vi "判斷輸贏.vi"(2 "フ":bool[][](array[boolean]), 3 "黑":bool[][](array[boolean])) -> (0 "フ墓":bool, 1 "黑贏":bool)   [LabVIEW 2014]
panel:
  out "黑贏(右上斜)":bool
  out "白贏(右上斜)":bool
  out "白贏(右下斜)":bool
  out "黑贏(右下斜)":bool
  out "フ墓(row)":bool
  out "フ墓(column)":bool
  out "黑贏(row)":bool
  out "黑贏(column)":bool
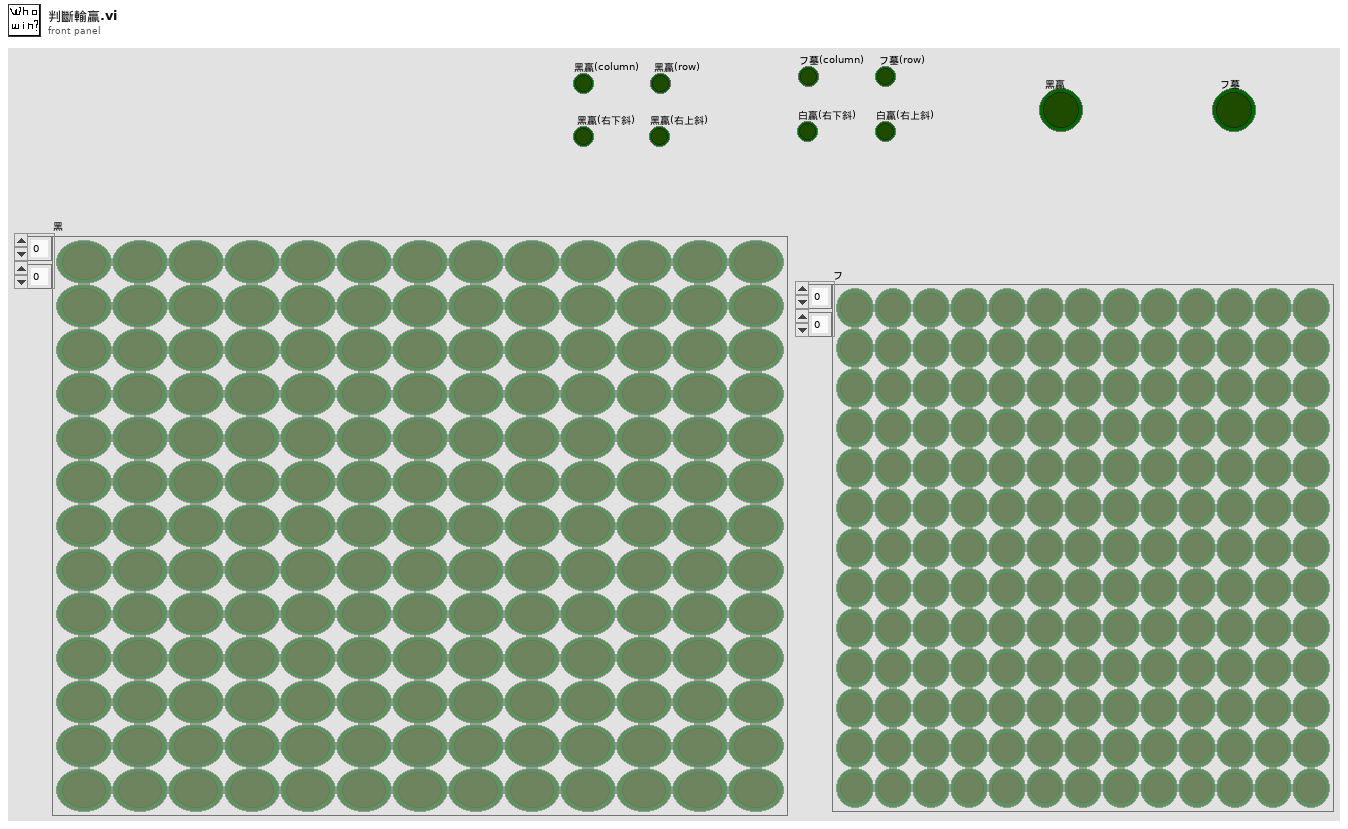
[diagram p1: front panel]
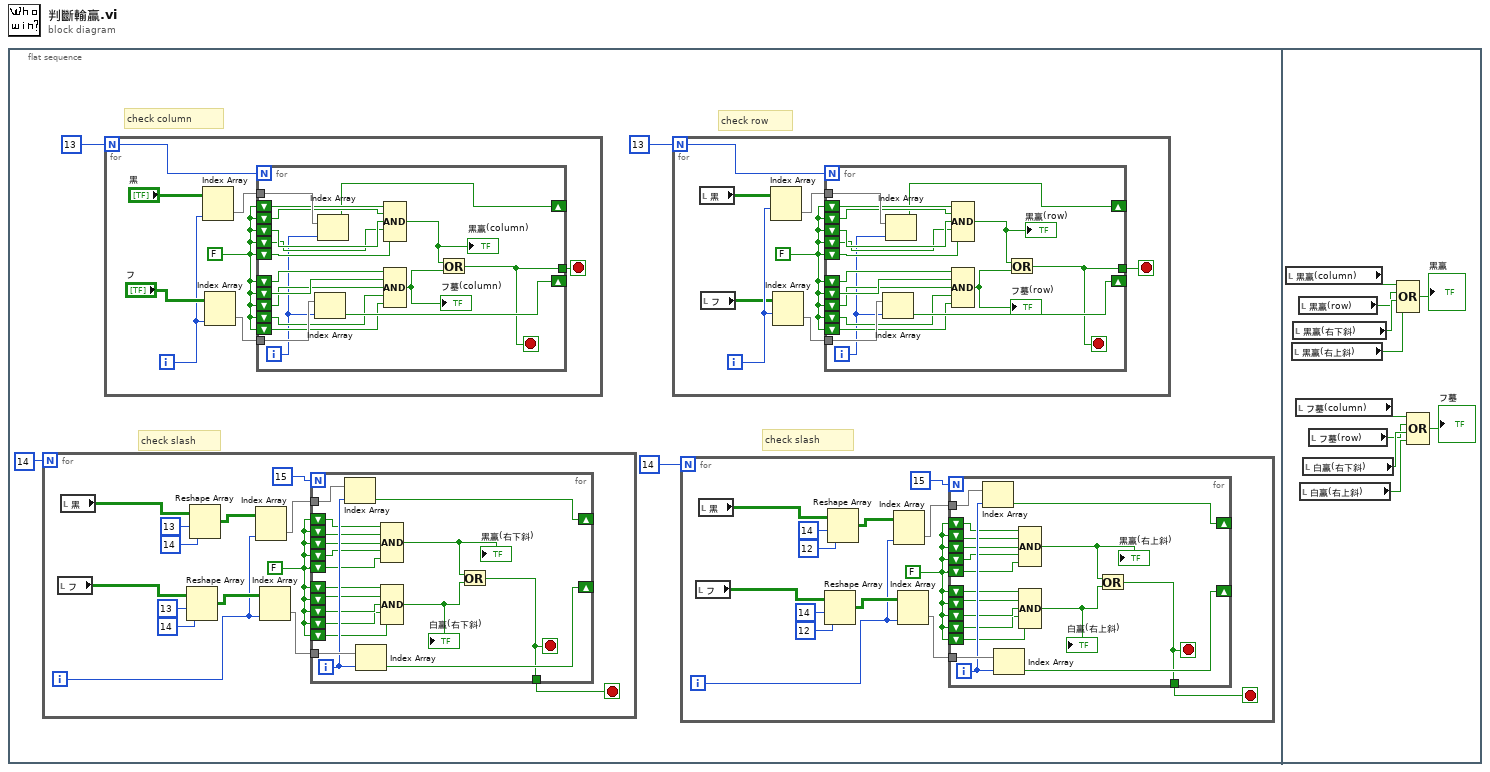
[diagram p0: block diagram]
diagram:
  n1 = flat-sequence {
    frame #0 {
      # "check slash"
      # "check slash"
      # "check row"
      # "check column"
      n2 = for {
        N: 14 -> [_]
        i -> [w42]
        stop <- w38 stop-if-true
        w39 = FALSE
        n3 = local read "フ"() -> (w48:bool[][])
        n4 = local read "黑"() -> (w47:bool[][])
        n5 = Reshape Array(w48, 13 ("dimension size"), 14 ("dimension size")) -> (w43:bool[][])
        n6 = Reshape Array(w47, 13 ("dimension size"), 14 ("dimension size")) -> (w44:bool[][])
        n7 = Index Array(array=w44, index (col)=w42) -> (element=w41:bool[])  [unwired: 1 in]
        n8 = Index Array(array=w43, index (col)=w42) -> (element=w40:bool[])  [unwired: 1 in]
        n9 = for {
          N: 15 -> [_]
          tunnel: w41 -> [w68]
          tunnel: w40 -> [w66]
          shift-right: [w67] -> _
          shift-left: w39 -> [w62]
          shift-left: w39 -> [w61]
          shift-left: w39 -> [w60]
          shift-left: w39 -> [w58]
          shift-left: w39 -> [w59]
          shift-right: [w64] -> _
          shift-left: w39 -> [w56]
          shift-left: w39 -> [w55]
          shift-left: w39 -> [w54]
          shift-left: w39 -> [w53]
          shift-left: w39 -> [w52]
          tunnel: [w63] -> w38
          i -> [w65]
          stop <- w63 stop-if-true
          n10 = Index Array(array=w68, index=w65) -> (element=w67:bool)
          n11 = Index Array(array=w66, index=w65) -> (element=w64:bool)
          n12 = Compound Arithmetic op=AND(w62, w61, w60, w59, w58) -> (w57:bool)
          "黑贏(右下斜)" <- w57
          n13 = Compound Arithmetic op=AND(w56, w55, w54, w53, w52) -> (w51:bool)
          "白贏(右下斜)" <- w51
          n14 = Or(x=w57, y=w51) -> (x .or. y?=w63:bool)
        }
      }
      n15 = for {
        N: 13 -> [w101]
        i -> [w98]
        stop <- w95 stop-if-true
        w97 = FALSE
        n16 = Index Array(array="黑", index (col)=w98) -> (element=w100:bool[])  [unwired: 1 in]
        n17 = Index Array(array="フ", index (col)=w98) -> (element=w96:bool[])  [unwired: 1 in]
        n18 = for {
          N: w101 -> [_]
          tunnel: w100 -> [w120]
          shift-right: [w114] -> _
          shift-left: w97 -> [w119]
          shift-left: w97 -> [w118]
          shift-left: w97 -> [w117]
          shift-left: w97 -> [w116]
          shift-left: w97 -> [w115]
          shift-right: [w112] -> _
          shift-left: w97 -> [w111]
          shift-left: w97 -> [w110]
          shift-left: w97 -> [w108]
          shift-left: w97 -> [w107]
          shift-left: w97 -> [w109]
          tunnel: w96 -> [w113]
          tunnel: [w104] -> w95
          i -> [w103]
          stop <- w104 stop-if-true
          n19 = Index Array(array=w113, index=w103) -> (element=w112:bool)
          n20 = Index Array(array=w120, index=w103) -> (element=w114:bool)
          n21 = Compound Arithmetic op=AND(w119, w118, w117, w116, w115) -> (w106:bool)
          "黑贏(column)" <- w106
          n22 = Compound Arithmetic op=AND(w111, w110, w109, w108, w107) -> (w105:bool)
          "フ墓(column)" <- w105
          n23 = Or(x=w106, y=w105) -> (x .or. y?=w104:bool)
        }
      }
      n24 = for {
        N: 13 -> [w76]
        i -> [w71]
        stop <- w72 stop-if-true
        w74 = FALSE
        n25 = local read "黑"() -> (w70:bool[][])
        n26 = local read "フ"() -> (w69:bool[][])
        n27 = Index Array(array=w70, index (row)=w71) -> (element=w75:bool[])  [unwired: 1 in]
        n28 = Index Array(array=w69, index (row)=w71) -> (element=w73:bool[])  [unwired: 1 in]
        n29 = for {
          N: w76 -> [_]
          tunnel: w75 -> [w94]
          shift-right: [w88] -> _
          shift-left: w74 -> [w93]
          shift-left: w74 -> [w92]
          shift-left: w74 -> [w91]
          shift-left: w74 -> [w90]
          shift-left: w74 -> [w89]
          shift-right: [w86] -> _
          shift-left: w74 -> [w85]
          shift-left: w74 -> [w84]
          shift-left: w74 -> [w82]
          shift-left: w74 -> [w81]
          shift-left: w74 -> [w83]
          tunnel: w73 -> [w87]
          tunnel: [w78] -> w72
          i -> [w77]
          stop <- w78 stop-if-true
          n30 = Index Array(array=w87, index=w77) -> (element=w86:bool)
          n31 = Index Array(array=w94, index=w77) -> (element=w88:bool)
          n32 = Compound Arithmetic op=AND(w93, w92, w91, w90, w89) -> (w80:bool)
          "黑贏(row)" <- w80
          n33 = Compound Arithmetic op=AND(w85, w84, w83, w82, w81) -> (w79:bool)
          "フ墓(row)" <- w79
          n34 = Or(x=w80, y=w79) -> (x .or. y?=w78:bool)
        }
      }
      n35 = for {
        N: 14 -> [_]
        i -> [w10]
        stop <- w6 stop-if-true
        w7 = FALSE
        n36 = local read "フ"() -> (w16:bool[][])
        n37 = local read "黑"() -> (w15:bool[][])
        n38 = Reshape Array(w16, 14 ("dimension size"), 12 ("dimension size")) -> (w11:bool[][])
        n39 = Reshape Array(w15, 14 ("dimension size"), 12 ("dimension size")) -> (w12:bool[][])
        n40 = Index Array(array=w12, index (col)=w10) -> (element=w9:bool[])  [unwired: 1 in]
        n41 = Index Array(array=w11, index (col)=w10) -> (element=w8:bool[])  [unwired: 1 in]
        n42 = for {
          N: 15 -> [_]
          tunnel: w9 -> [w36]
          tunnel: w8 -> [w34]
          shift-right: [w35] -> _
          shift-left: w7 -> [w30]
          shift-left: w7 -> [w29]
          shift-left: w7 -> [w28]
          shift-left: w7 -> [w26]
          shift-left: w7 -> [w27]
          shift-right: [w32] -> _
          shift-left: w7 -> [w24]
          shift-left: w7 -> [w23]
          shift-left: w7 -> [w22]
          shift-left: w7 -> [w21]
          shift-left: w7 -> [w20]
          tunnel: [w31] -> w6
          i -> [w33]
          stop <- w31 stop-if-true
          n43 = Index Array(array=w36, index=w33) -> (element=w35:bool)
          n44 = Index Array(array=w34, index=w33) -> (element=w32:bool)
          n45 = Compound Arithmetic op=AND(w30, w29, w28, w27, w26) -> (w25:bool)
          "黑贏(右上斜)" <- w25
          n46 = Compound Arithmetic op=AND(w24, w23, w22, w21, w20) -> (w19:bool)
          "白贏(右上斜)" <- w19
          n47 = Or(x=w25, y=w19) -> (x .or. y?=w31:bool)
        }
      }
    }
    frame #1 {
      n48 = local read "黑贏(column)"() -> (w121:bool)
      n49 = local read "黑贏(右上斜)"() -> (w130:bool)
      n50 = local read "黑贏(右下斜)"() -> (w127:bool)
      n51 = local read "フ墓(column)"() -> (w126:bool)
      n52 = local read "黑贏(row)"() -> (w122:bool)
      n53 = local read "白贏(右上斜)"() -> (w129:bool)
      n54 = local read "白贏(右下斜)"() -> (w128:bool)
      n55 = local read "フ墓(row)"() -> (w125:bool)
      n56 = Compound Arithmetic op=OR(w121, w122, w127, w130) -> (→"黑贏":bool)
      n57 = Compound Arithmetic op=OR(w126, w125, w128, w129) -> (→"フ墓":bool)
    }
  }
